vi "EXPERIMENTAL_RECONFIGURE_DCPOWERCARDS.vi"() -> ()   [LabVIEW 2019]
uses:
  Controls/DCPowerBlock_byChannel_Control.ctl
  Controls/PlotColorArray.ctl
panel:
  out "Current Numeric (A)":dbl[][](array[numeric])
  out "Voltage Numeric (V)":dbl[][](array[numeric])
  out "Current Waveform Array":waveform(dbl)[](graph)
  out "Voltage Waveform Array":waveform(dbl)[](graph)
  out "DCPowerInformationClusterArray":T1(array[cluster])
  in  "error in":errorcluster
  in  "DCPowerInformation_byChannel_input":T2(array[cluster])
  out "DCPowerInformation_byChannel_output":T2(array[cluster])
  out "error out":errorcluster
  in  "ColorPalette":T3=[16711686, 65351, 8978420, 14474240, 16139007, 16752640, 8958719, 16758973, 16777215, 46792, 11992992, 12961221, 16763690, 12600063, 16711835, 2953983, 40796, 13111296, 13352613, 9221011, 12964076, 12819897, 65442, 16776704, 14540253, 16740729, 10658047, 10813344, 16753521, 13413843, 8691115, 10339240, 14401205, 16746704, 7467519, 16775978, 13872558, 11387603, 13354405, 10420227, 13107364, 4060, 35208, 11817216, 7566080, 40796, 7539456, 2837073, 6372186, 7499083, 10648702, 16757152]
  in  "DC Power Block Configuration":T4
  in  "power channel select":u16(ring) items=["Slot_4_PXIe4139channel number:  0; channel name: Red 5v", "Slot_5_PXIe4139channel number:  0; channel name: Orange 3.3v_6780", "Slot_6_PXIe4139channel number:  0; channel name: Yellow 1.8v", "PXIe4163channel number:  0; channel name: Green 3.3v", "PXIe4163channel number:  1; channel name: Blue 2.6v VATT"]
  in  "setting change select":u16(ring) items=["voltage", "channel name"]
  in  "Apply Change":bool
  in  "End Reconfig":bool
  # "Nothing to see behind here, surely"
  # "THESE ARE THE ONLY TWO YOU CAN UPDATE ON THIS RING. CHANNEL NUMBER TO BE ADDED AS NEEDED/REQUESTED"
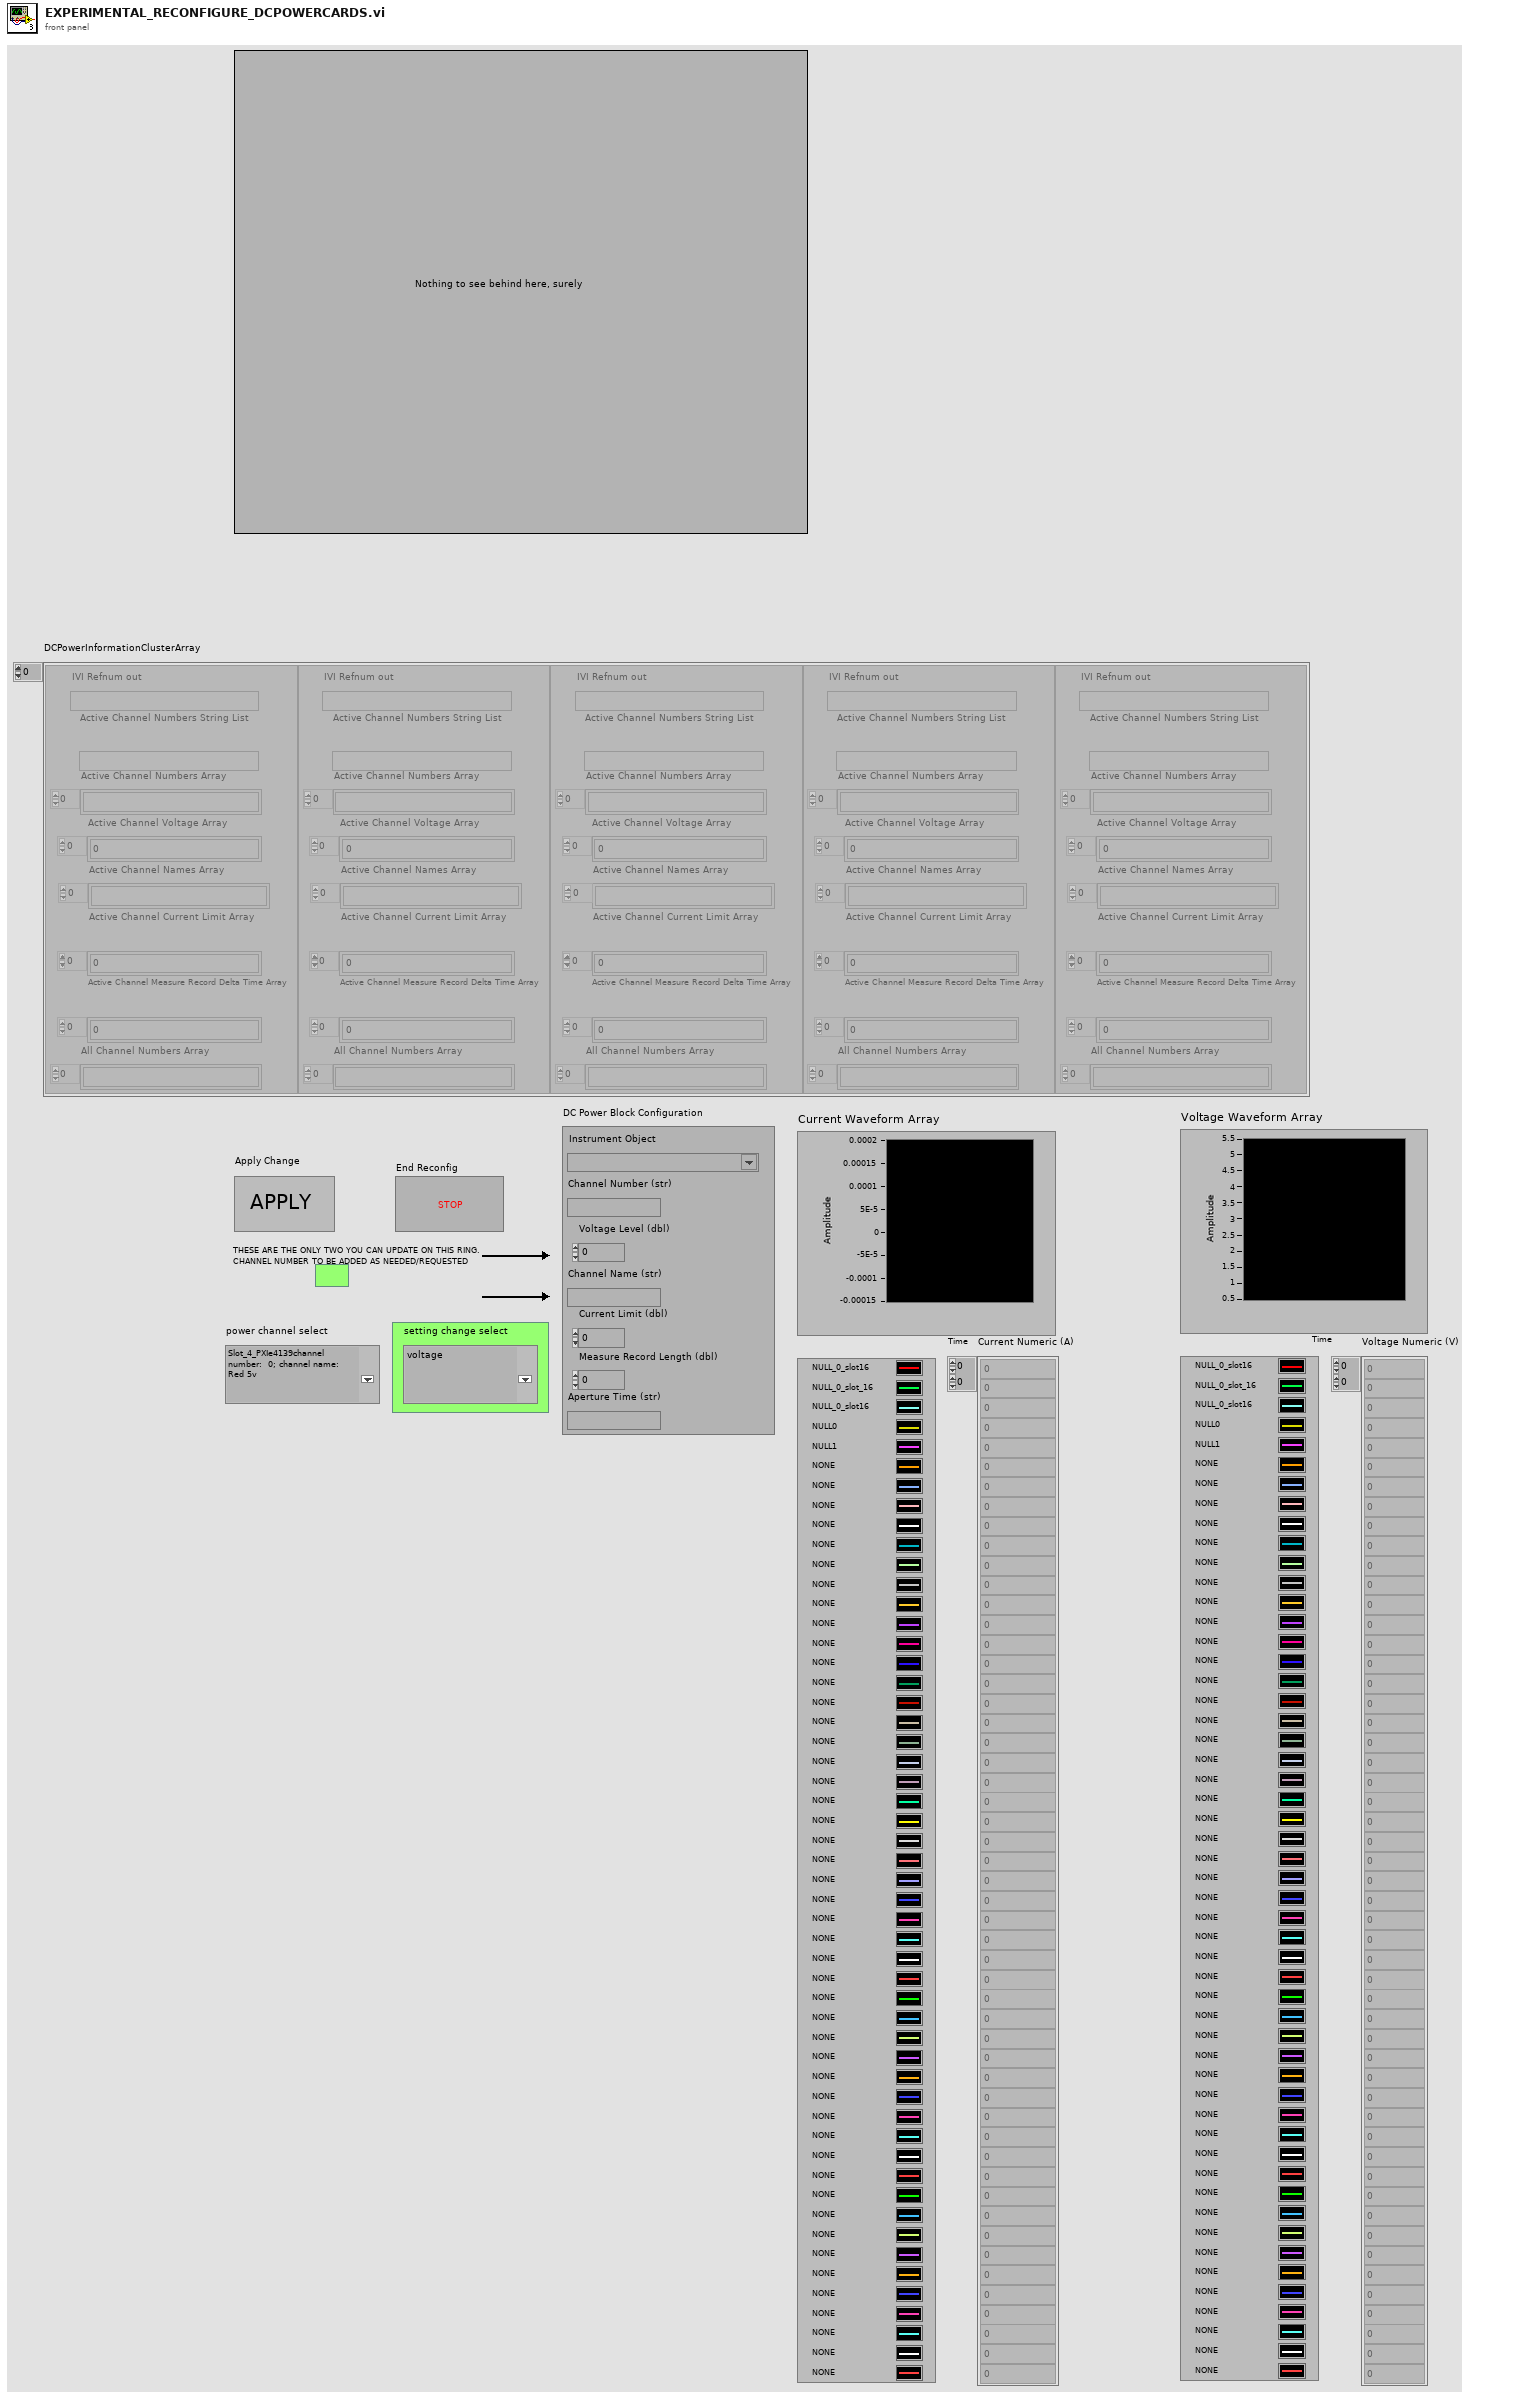
[diagram p1: front panel]
types:
  T1 = cluster{"IVI Refnum out":refnum<k15>, "Active Channel Numbers String List":string, "Active Channel Numbers Array":string[], "Active Channel Voltage Array":dbl[], "Active Channel Names Array":string[], "Active Channel Current Limit Array":dbl[], "Active Channel Measure Record Delta Time Array":dbl[], "All Channel Numbers Array":string[]}[]
  T2 = cluster{"IVI Refnum out":refnum<k15>, string, "voltage level channel 23":dbl, "Channel Name 23":string, "Current Limit":dbl, "Measure Record dt":dbl, string}[]
  T3 = typedef "PlotColorArray.ctl" = u32[]
  T4 = typedef "DCPowerBlock_byChannel_Control.ctl" = cluster{"Instrument Object":refnum<k15>, "Channel Number (str)":string, "Voltage Level (dbl)":dbl, "Channel Name (str)":string, "Current Limit (dbl)":dbl, "Measure Record Length (dbl)":dbl, "Aperture Time (str)":string}
  T5 = typedef "LVStringsAndValuesArrayTypeDef_U16.ctl" = cluster{"String":string, "Value":u16}[]
  T6 = cluster{"IVI Refnum out":refnum<k15>, string, "voltage level channel 23":dbl, "Channel Name 23":string, "Current Limit":dbl, "Measure Record dt":dbl, string}
  T7 = cluster{"instrument handle out":refnum<k15>, string, "Voltage Level (dbl)":dbl, "Channel Name 23":string, "Current Limit":dbl, "Measure Record dt":dbl, string}
  T8 = cluster{"IVI Refnum out":refnum<k15>, string, "voltage level channel 23":dbl, "Channel Name (str)":string, "Current Limit":dbl, "Measure Record dt":dbl, string}
  T9 = cluster{"IVI Refnum out":refnum<k15>, "String List":string, string[], dbl[], string[], dbl[], dbl[], string[]}[]
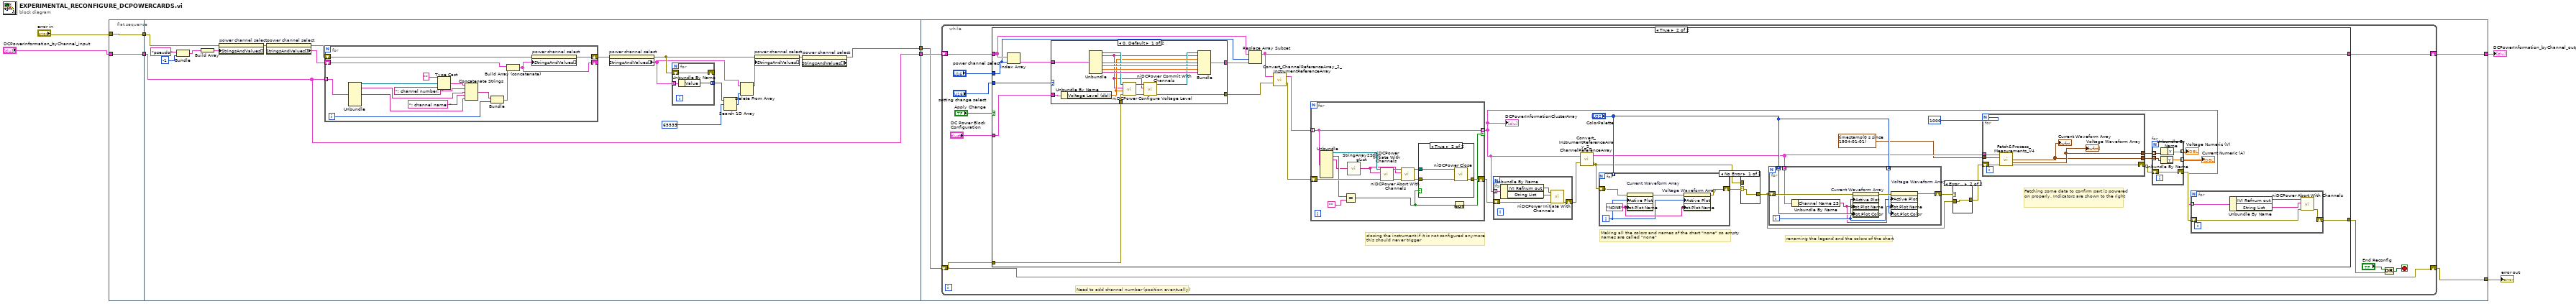
[diagram p0: block diagram]
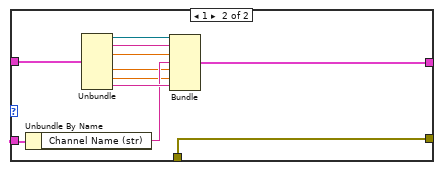
[diagram p6: hidden frame]
diagram:
  n1 = flat-sequence {
    tunnel: "DCPowerInformation_byChannel_input" -> [w10]
    tunnel: [w10] -> w8
    tunnel: [w9] -> w7
    tunnel: "error in" -> [w9]
    tunnel: w8 -> [w12]
    tunnel: w7 -> [w25]
    tunnel: [w12] -> w6
    tunnel: [w11] -> w5
    tunnel: w6 -> [w50]
    tunnel: w5 -> [w49]
    tunnel: [w48] -> w4
    tunnel: [w47] -> w3
    frame #0 {
    }
    frame #1 {
      n2 = Bundle("concatenated string"="pseudo", -1) -> (w24:cluster{"concatenated string":string, i32})  [unwired: 1 in]
      n3 = Build Array(w24) -> (w23:cluster{"concatenated string":string, i32}[])
      n4 = property on="power channel select" class="Ring (strict)"(error in=w25, "StringsAndValues[]"=w23) -> (error out=w26:errorcluster)  [unwired: 1 in, 1 out]
      n5 = property on="power channel select" class="Ring (strict)"(error in=w26) -> (error out=w27:errorcluster, "StringsAndValues[]"=w28:T5)  [unwired: 1 in, 1 out]
      n6 = for {
        tunnel: w12 -> [w37] mode=indexing
        shift-right: [w32] -> _
        shift-left: w28 -> [w34]
        shift-right: [w35] -> w20
        shift-left: w27 -> [w46]
        i -> [w36]
        n7 = Unbundle(w37) -> ("IVI Refnum out"=w45:refnum<k15>, w41:string, "Channel Name 23"=w39:string)  [unwired: 4 out]
        n8 = Type Cast(type="", x=w45) -> (*(type *) &x=w43:string)
        n9 = Concatenate Strings(w43, "; channel number:  " ("string"), w41, "; channel name: " ("string"), w39) -> (w38:string)
        n10 = Bundle(w38, w36) -> (w33:cluster{string, i32})  [unwired: 1 in]
        n11 = Build Array (concatenate)(w34, w33) -> (w32:cluster{"String":string, "Value":i32}[])
        n12 = property on="power channel select" class="Ring (strict)"(error in=w46, "StringsAndValues[]"=w32) -> (error out=w35:errorcluster)  [unwired: 1 in, 1 out]
      }
      n13 = property on="power channel select" class="Ring (strict)"(error in=w20) -> (error out=w19:errorcluster, "StringsAndValues[]"=w15:T5)  [unwired: 1 in, 1 out]
      n14 = for {
        tunnel: w15 -> [w31] mode=indexing
        shift-right: [w29] -> _
        shift-left: w19 -> [w29]
        tunnel: [w30] -> w17 mode=indexing
        n15 = Unbundle By Name(w31) -> ("Value"=w30:u16)
      }
      n16 = Search 1D Array(1D array=w17, element=u16 65535) -> (index of element=w18:i32)  [unwired: 1 in]
      n17 = Delete From Array(array=w15, index=w18) -> (array with subset deleted=w14:T5)  [unwired: 1 in, 1 out]
      n18 = property on="power channel select" class="Ring (strict)"(error in=w19, "StringsAndValues[]"=w14) -> (error out=w13:errorcluster)  [unwired: 1 in, 1 out]
      n19 = property on="power channel select" class="Ring (strict)" props=["StringsAndValues[]"](error in=w13) -> (error out=w11:errorcluster)  [unwired: 1 in, 2 out]
    }
    frame #2 {
      n20 = while {
        shift-right: [w56] -> w47
        shift-left: w50 -> [w58]
        shift-right: [w52] -> w48
        shift-left: w49 -> [w52]
        stop <- w55 stop-if-true
        # "Need to add channel number (position eventually)"
        n21 = case shown="True" "Apply Change" {
          tunnel: "power channel select" -> [_ w87]
          tunnel: w58 -> [w62 w89]
          tunnel: "DC Power Block Configuration" -> [_ w91]
          tunnel: "setting change select" -> [_ w92]
          tunnel: [w62 w85] -> w56
          tunnel: w52 -> [w61 w86]
          tunnel: [w61 w64] -> w51
          frame False {
          }
          frame True {
            # "Fetching some data to confirm part is powered on properly. Indicators are shown to the right"
            # "Making all the colors and names of the chart \"none\" so empty names are called \"none\""
            # "renaming the legend and the colors of the chart"
            # "closing the instrument if it is not configured anymore\nthis should never trigger"
            n22 = Index Array(array=w89, index=w87) -> (element=w90:T6)
            n23 = case shown="0, Default" w92 {
              tunnel: w91 -> [w157 w174]
              tunnel: w90 -> [w160 w173]
              tunnel: [w158 w165] -> w88
              tunnel: w86 -> [w156 w164]
              tunnel: [w151 w164] -> w65
              frame 0, Default {
                n24 = Unbundle By Name(w157) -> ("Voltage Level (dbl)"=w154:dbl)
                n25 = Unbundle(w160) -> ("IVI Refnum out"=w155:refnum<k15>, w149:string, "Channel Name 23"=w159:string, "Current Limit"=w162:dbl, "Measure Record dt"=w161:dbl, w163:string)  [unwired: 1 out]
                n26 = call <instrlib>:"niDCPower Configure Voltage Level.vi"("error in (no error)"=w156, "voltage level"=w154, "channel name"=w149, "instrument handle"=w155) -> ("error out"=w153:errorcluster, "instrument handle out"=w152:refnum<k15>)  [unwired: 6 in]
                n27 = call <instrlib>:"niDCPower Commit With Channels.vi"("error in (no error)"=w153, "channel name"=w149, "instrument handle"=w152) -> ("error out"=w151:errorcluster, "instrument handle out"=w150:refnum<k15>)  [unwired: 7 in]
                n28 = Bundle("instrument handle out"=w150, w149, "Voltage Level (dbl)"=w154, "Channel Name 23"=w159, "Current Limit"=w162, "Measure Record dt"=w161, w163) -> (w158:T7)  [unwired: 1 in]
              }
              frame 1 {
                n29 = Unbundle By Name(w174) -> ("Channel Name (str)"=w168:string)
                n30 = Unbundle(w173) -> ("IVI Refnum out"=w172:refnum<k15>, w170:string, "voltage level channel 23"=w169:dbl, "Current Limit"=w167:dbl, "Measure Record dt"=w166:dbl, w171:string)  [unwired: 1 out]
                n31 = Bundle("IVI Refnum out"=w172, w170, "voltage level channel 23"=w169, "Channel Name (str)"=w168, "Current Limit"=w167, "Measure Record dt"=w166, w171) -> (w165:T8)  [unwired: 1 in]
              }
            }
            n32 = Replace Array Subset(array=w89, new element=w88, index=w87) -> (w85:T2)
            n33 = call "Convert_ChannelReferenceArray_2_InstrumentReferenceArray.vi"("error in"=w65, "DCPowerInformation_byChannel"=w85) -> ("error out"=w63:errorcluster, "Array"=w66:T9)
            n34 = for {
              tunnel: [w144] -> w75 mode=indexing if=w133
              tunnel: w66 -> [w144] mode=indexing
              shift-right: [w135] -> w70
              shift-left: w63 -> [w142]
              n35 = Unbundle(w144) -> ("IVI Refnum out"=w143:refnum<k15>, "String List"=w138:string, w131:string[])  [unwired: 5 out]
              n36 = Equal?(x=w138, y="") -> (x = y?=w134:bool)
              n37 = call "StringArray2StringList.vi"("String Array"=w131) -> ("String List"=w137:string)
              n38 = call <instrlib>:"niDCPower Initiate With Channels.vi"("error in (no error)"=w142, "channel name"=w137, "instrument handle"=w143) -> ("error out"=w141:errorcluster, "instrument handle out"=w140:refnum<k15>)  [unwired: 7 in]
              n39 = call <instrlib>:"niDCPower Abort With Channels.vi"("error in (no error)"=w141, "channel name"=w137, "instrument handle"=w140) -> ("error out"=w136:errorcluster, "instrument handle out"=w132:refnum<k15>)  [unwired: 7 in]
              n40 = case shown="True" w134 {
                tunnel: w136 -> [w145 w148]
                tunnel: [w145 w146] -> w135
                tunnel: w132 -> [_ w147]
                frame False {
                }
                frame True {
                  n41 = call <instrlib>:"niDCPower Close.vi"("error in (no error)"=w148, "instrument handle"=w147) -> ("error out"=w146:errorcluster)  [unwired: 9 in]
                }
              }
              n42 = Not(x=w134) -> (.not. x?=w133:bool)
            }
            "DCPowerInformationClusterArray" <- w75
            n43 = for {
              tunnel: w75 -> [w130] mode=indexing
              shift-right: [w127] -> w69
              shift-left: w70 -> [w126]
              n44 = Unbundle By Name(w130) -> ("IVI Refnum out"=w128:refnum<k15>, "String List"=w129:string)
              n45 = call <instrlib>:"niDCPower Initiate With Channels.vi"("error in (no error)"=w126, "channel name"=w129, "instrument handle"=w128) -> ("error out"=w127:errorcluster)  [unwired: 7 in, 1 out]
            }
            n46 = call "Convert_InstrumentReferenceArray_2_ChannelReferenceArray.vi"("error in (no error)"=w69, "DCPowerInformationClusterArray_Input"=w75) -> ("error out"=w72:errorcluster, "DCPowerInformation_byChannel"=w73:T2)
            n47 = for {
              shift-right: [w119] -> w71
              shift-left: w72 -> [w117]
              tunnel: "ColorPalette" -> [_] mode=indexing
              i -> [w116]
              w115 = "NONE" ("Plot.Plot Name")
              n48 = property on="Current Waveform Array" class="WFChart (strict)"(error in=w117, "Active Plot"=w116, "Plot.Plot Name"=w115) -> (error out=w118:errorcluster)  [unwired: 1 in, 1 out]
              n49 = property on="Voltage Waveform Array" class="WFChart (strict)"(error in=w118, "Active Plot"=w116, "Plot.Plot Name"=w115) -> (error out=w119:errorcluster)  [unwired: 1 in, 1 out]
            }
            n50 = case shown="No Error" w71 {
              selector: w71 -> [w113 _]
              tunnel: [w113 w114] -> w77
              tunnel: w72 -> [_ w114]
              frame No Error {
              }
              frame Error {
              }
            }
            n51 = for {
              shift-right: [w110] -> w78
              shift-left: w77 -> [w111]
              tunnel: w73 -> [w109] mode=indexing
              tunnel: "ColorPalette" -> [w108] mode=indexing
              tunnel: "ColorPalette" -> [w107] mode=indexing
              i -> [w106]
              n52 = Unbundle By Name(w109) -> ("Channel Name 23"=w105:string)
              n53 = property on="Current Waveform Array" class="WFChart (strict)"(error in=w111, "Active Plot"=w106, "Plot.Plot Name"=w105, "Plot.Plot Color"=w108) -> (error out=w112:errorcluster)  [unwired: 1 in, 1 out]
              n54 = property on="Voltage Waveform Array" class="WFChart (strict)"(error in=w112, "Active Plot"=w106, "Plot.Plot Name"=w105, "Plot.Plot Color"=w107) -> (error out=w110:errorcluster)  [unwired: 1 in, 1 out]
            }
            n55 = case shown="Error .." w78 {
              selector: w78 -> [w98 _]
              tunnel: [w98 w99] -> w76
              tunnel: w77 -> [_ w99]
              frame No Error {
              }
              frame Error {
              }
            }
            n56 = for {
              N: 1000 -> [_]
              tunnel: w73 -> [w125]
              tunnel: timestamp(0 s since 1904-01-01) ("Initial Time") -> [w124]
              shift-right: [w122] -> w81
              shift-left: w76 -> [w123]
              tunnel: [w121] -> w79
              tunnel: [w120] -> w82
              n57 = call "Fetch&Process_Measurements_V4.vi"("DCPowerInformation_byChannel"=w125, "Initial Time"=w124, "error in (no error)"=w123) -> ("Current Waveform Array"=w120:waveform(dbl)[], "Voltage Waveform Array"=w121:waveform(dbl)[], "error out"=w122:errorcluster)  [unwired: 6 in, 4 out]
              "Current Waveform Array" <- w120
              "Voltage Waveform Array" <- w121
            }
            n58 = for {
              tunnel: w79 -> [w97] mode=indexing
              shift-right: [w96] -> w80
              shift-left: w81 -> [w96]
              tunnel: w82 -> [w95] mode=indexing
              tunnel: [w94] -> w83 mode=indexing
              tunnel: [w93] -> w84 mode=indexing
              n59 = Unbundle By Name(w95) -> ("Y"=w93:dbl[])
              n60 = Unbundle By Name(w97) -> ("Y"=w94:dbl[])
            }
            "Voltage Numeric (V)" <- w83
            "Current Numeric (A)" <- w84
            n61 = for {
              tunnel: w75 -> [w104] mode=indexing
              shift-right: [w100] -> w64
              shift-left: w80 -> [w101]
              n62 = Unbundle By Name(w104) -> ("IVI Refnum out"=w103:refnum<k15>, "String List"=w102:string)
              n63 = call <instrlib>:"niDCPower Abort With Channels.vi"("error in (no error)"=w101, "channel name"=w102, "instrument handle"=w103) -> ("error out"=w100:errorcluster)  [unwired: 7 in, 1 out]
            }
          }
        }
        n64 = Or(x="End Reconfig", y=w51) -> (x .or. y?=w55:bool)
      }
    }
  }
  "error out" <- w4
  "DCPowerInformation_byChannel_output" <- w3
